vi "VCI_StartCAN.vi"(9 "CANIndex":u32, 10 "DevIndex":u32, 11 "DevType":u32) -> (1 "CANIndex 2":u32, 2 "DevIndex 2":u32, 3 "DevType 2":u32, 5 "StartCAN_Success?":u32)   [LabVIEW 2014]
uses:
  ControlCAN.dll
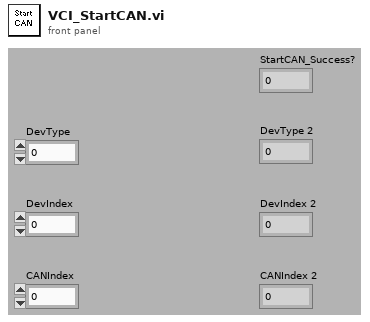
[diagram p1: front panel]
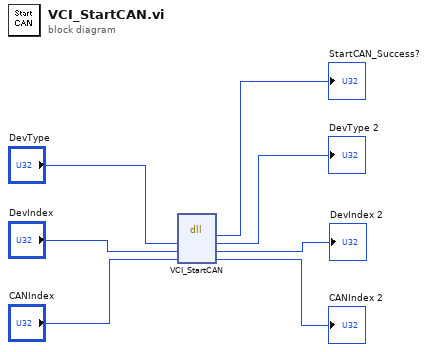
[diagram p0: block diagram]
diagram:
  n1 = dll-call lib="D:/Documents/USBCAN/USBCAN/ControlCAN.dll" fn="VCI_StartCAN"("DevType"="DevType", "DevIndex"="DevIndex", "CANIndex"="CANIndex") -> ("StartCAN_Success?"=→"StartCAN_Success?":u32, "DevType"=→"DevType 2":u32, "DevIndex"=→"DevIndex 2":u32, "CANIndex"=→"CANIndex 2":u32)  [unwired: 3 in, 2 out]
